vi "tiff test.vi"(0 "Image In":T1, 2 "Target File Path":path, 5 "Max":i32, 7 "Min":i32, 11 "Error in (no error)":errorcluster) -> (4 "Image":T1(plugin-control), 15 "Error out":errorcluster)   [LabVIEW 2021]
uses:
  <vilib>/vision/Image Controls.llb/IMAQ Image.ctl
  <vilib>/vision/NI_Vision_Development_Module.lvlib
panel:
  in  "File Path In":path
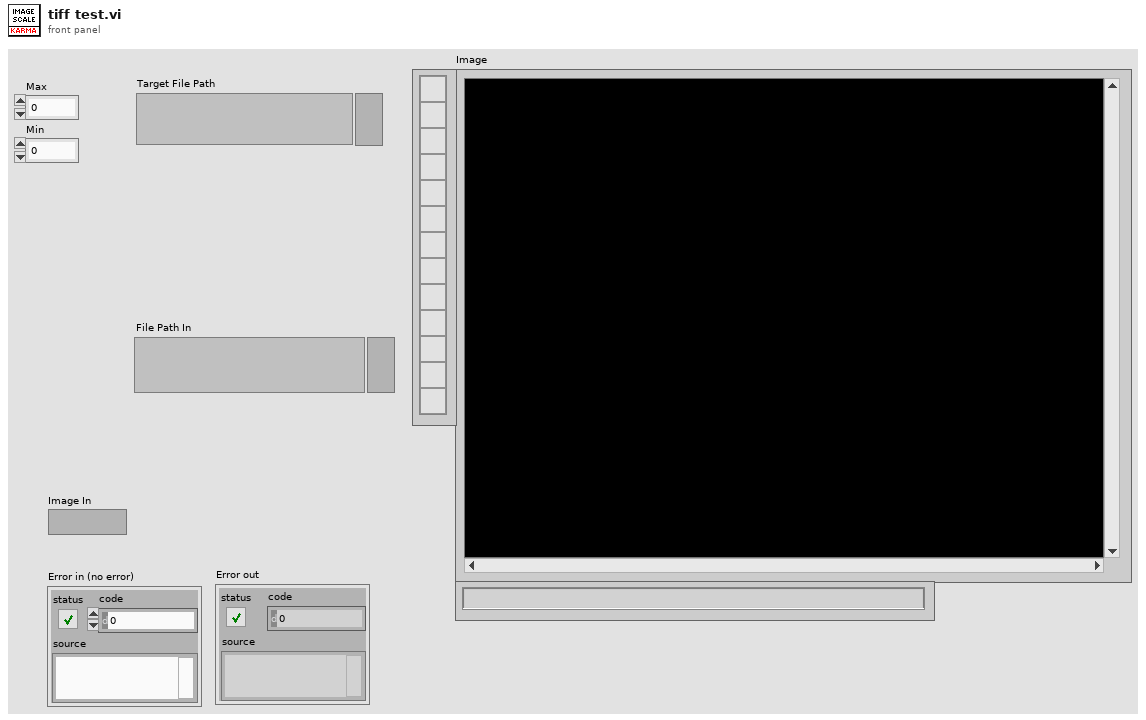
[diagram p1: front panel]
types:
  T1 = typedef "IMAQ Image.ctl" = refnum<image>
  T2 = typedef "Image Type" = u32
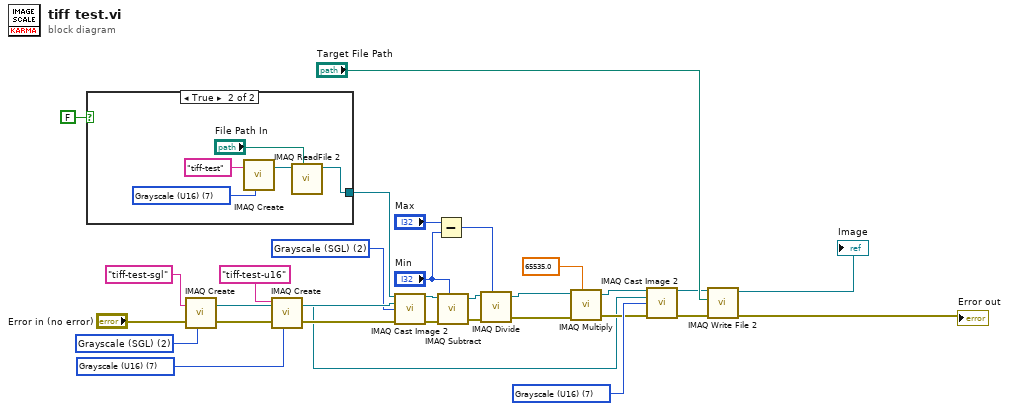
[diagram p0: block diagram]
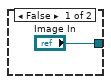
[diagram p2: hidden frame]
diagram:
  w4 = T2 7 items=["Grayscale (U8)", "Grayscale (I16)", "Grayscale (SGL)", "Complex (CSG)", "RGB (U32)", "HSL (U32)", "RGB (U64)", "Grayscale (U16)"] ("Image Type")
  w18 = T2 7 items=["Grayscale (U8)", "Grayscale (I16)", "Grayscale (SGL)", "Complex (CSG)", "RGB (U32)", "HSL (U32)", "RGB (U64)", "Grayscale (U16)"] ("Image Type")
  w21 = T2 2 items=["Grayscale (U8)", "Grayscale (I16)", "Grayscale (SGL)", "Complex (CSG)", "RGB (U32)", "HSL (U32)", "RGB (U64)", "Grayscale (U16)"] ("Image Type")
  w24 = T2 2 items=["Grayscale (U8)", "Grayscale (I16)", "Grayscale (SGL)", "Complex (CSG)", "RGB (U32)", "HSL (U32)", "RGB (U64)", "Grayscale (U16)"] ("Image Type")
  n1 = case shown="True" FALSE {
    tunnel: ["Image In" w32] -> w14
    frame False {
    }
    frame True {
      w35 = T2 7 items=["Grayscale (U8)", "Grayscale (I16)", "Grayscale (SGL)", "Complex (CSG)", "RGB (U32)", "HSL (U32)", "RGB (U64)", "Grayscale (U16)"] ("Image Type")
      n2 = call "IMAQ Create"("Image Name"="tiff-test", "Image Type"=w35) -> ("New Image"=w33:T1)  [unwired: 3 in, 1 out]
      n3 = call "IMAQ ReadFile 2"("File Path"="File Path In", "Image"=w33) -> ("Image Out"=w32:T1)  [unwired: 5 in, 4 out]
    }
  }
  n4 = call "IMAQ Create"("Image Name"="tiff-test-sgl", "Image Type"=w24, "error in (no error)"="Error in (no error)") -> ("New Image"=w22:T1, "error out"=w3:errorcluster)  [unwired: 2 in]
  n5 = call "IMAQ Create"("Image Name"="tiff-test-u16", "Image Type"=w4, "error in (no error)"=w3) -> ("New Image"=w1:T1, "error out"=w2:errorcluster)  [unwired: 2 in]
  n6 = call "IMAQ Cast Image 2"("Image Src"=w14, "Image Dst"=w22, "Image Type"=w21, "error in (no error)"=w2) -> ("Image Dst Out"=w25:T1, "error out"=w12:errorcluster)  [unwired: 10 in]
  n7 = Subtract(x="Max", y="Min") -> (x-y=w28:i32)
  n8 = call "IMAQ Subtract"("Image Src A"=w25, "Constant"="Min", "error in (no error)"=w12) -> ("Image Dst Out"=w29:T1, "error out"=w11:errorcluster)  [unwired: 4 in]
  n9 = call "IMAQ Divide"("Image Src A"=w29, "Constant"=w28, "error in (no error)"=w11) -> ("Image Dst Out"=w27:T1, "error out"=w10:errorcluster)  [unwired: 4 in]
  n10 = call "IMAQ Multiply"("Image Src A"=w27, "Constant"=65535.0, "error in (no error)"=w10) -> ("Image Dst Out"=w20:T1, "error out"=w9:errorcluster)  [unwired: 4 in]
  n11 = call "IMAQ Cast Image 2"("Image Src"=w20, "Image Dst"=w1, "Image Type"=w18, "error in (no error)"=w9) -> ("Image Dst Out"=w19:T1, "error out"=w8:errorcluster)  [unwired: 10 in]
  n12 = call-poly "IMAQ Write File 2"("error in (no error)"=w8, "File Path"="Target File Path", "Image"=w19) -> ("error out"=→"Error out":errorcluster, "Image Out (duplicate)"=→"Image":T1)  [unwired: 7 in]
